vi "HH_CalcBinningValues.vi"(11 "Bin Steps":i32) -> (3 "BinningValues":cluster{"String":string, "Value":i32}[](array[cluster]))   [LabVIEW 2017]
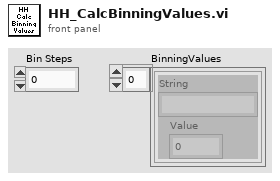
[diagram p1: front panel]
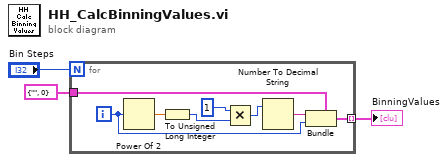
[diagram p0: block diagram]
diagram:
  n1 = for {
    N: "Bin Steps" -> [_]
    tunnel: cluster{"String":string, "Value":i32} {"String"="", "Value"=0} -> [w11]
    tunnel: [w4] -> w3 mode=indexing
    i -> [w10]
    n2 = Power Of 2(x=w10) -> (2^x=w9:dbl)
    n3 = To Unsigned Long Integer(number=w9) -> (unsigned 32bit integer=w8:u32)
    n4 = Multiply(x=u32 1, y=w8) -> (x*y=w6:u32)
    n5 = Number To Decimal String(number=w6) -> (decimal integer string=w5:string)  [unwired: 1 in]
    n6 = Bundle(cluster=w11, "String"=w5, "Value"=w10) -> (w4:cluster{"String":string, "Value":i32})
  }
  "BinningValues" <- w3
